vi "Finish.vi"   [LabVIEW 2015]
doc: "This VI is called just before exiting. It is expected to close I/O refnum, save collected data, etc."
uses:
  <vilib>/Rock Robotics/WPI/Utilities/WPI_GetSetVariantRefNum.vi
  navX Library v2/navX Library v2.lvlib
types:
  T1 = typedef "WPI_DigitalInputDevRef.ctl" = cluster{"DevStatus":errorcluster, "DIO Channel":T2}
  T2 = typedef "FPGA_DIOChannel.ctl" = enum8{"DIO 0", "DIO 1", "DIO 2", "DIO 3", "DIO 4", "DIO 5", "DIO 6", "DIO 7", "DIO 8", "DIO 9", "DIO MXP 0", "DIO MXP 1", "DIO MXP 2", "DIO MXP 3", "DIO MXP 4", "DIO MXP 5", "DIO MXP 6", "DIO MXP 7", "DIO MXP 8", "DIO MXP 9", "DIO MXP 10", "DIO MXP 11", "DIO MXP 12", "DIO MXP 13", "DIO MXP 14", "DIO MXP 15", "Invalid"}
  T3 = typedef "WPI_SolenoidDevRef.ctl" = cluster{"DevStatus":errorcluster, "Pneumatics Control Module":u8, "Forward Solenoid Channel":T4, "Reverse Solenoid Channel":T4}
  T4 = typedef "WPI_SolenoidChannel.ctl" = enum8{"Solenoid 0", "Solenoid 1", "Solenoid 2", "Solenoid 3", "Solenoid 4", "Solenoid 5", "Solenoid 6", "Solenoid 7", "Invalid"}
  T5 = typedef "WPI_AnalogChannelDevRef.ctl" = cluster{"DevStatus":errorcluster, "Analog Channel":T6}
  T6 = typedef "FPGA_AIChannel.ctl" = enum8{"AI 0", "AI 1", "AI 2", "AI 3", "AI MXP 0", "AI MXP 1", "AI MXP 2", "AI MXP 3", "Invalid"}
  T7 = typedef "WPI_MotorControlDeviceRef.ctl" = cluster{"DeviceStatus":errorcluster, "Type":T8, "PWM":cluster{"PWM Channel":T9, "DeadBand":T10}, "CAN":cluster{"Device Number":u8, "Control Mode":T11, "Semaphore":T12, "Max Vout":dbl, "TalonSRX Control Mode":T13}, "Invert":bool}
  T8 = typedef "WPI_MotorControlType.ctl" = enum16{"PWM", "CAN", "CANTalonSRX"}
  T9 = typedef "FPGA_DIOPWMChannel.ctl" = enum8{"PWM 0", "PWM 1", "PWM 2", "PWM 3", "PWM 4", "PWM 5", "PWM 6", "PWM 7", "PWM 8", "PWM 9", "PWM MXP 0", "PWM MXP 1", "PWM MXP 2", "PWM MXP 3", "PWM MXP 4", "PWM MXP 5", "PWM MXP 6", "PWM MXP 7", "PWM MXP 8", "PWM MXP 9", "Invalid"}
  T10 = typedef "WPI_PWMDeadband.ctl" = cluster{"Name":string, "maxPositivePwm":i32, "minPositivePwm":i32, "centerPwm":i32, "maxNegativePwm":i32, "minNegativePwm":i32, "angularRange":u16}
  T11 = typedef "WPI_CANJaguar_ControlMode.ctl" = enum8{"Percent VBus", "Current", "Speed", "Position", "Voltage"}
  T12 = typedef "Semaphore RefNum" = refnum<k1>
  T13 = typedef "WPI_CANTalonSRX_APIControlMode.ctl" = enum8{"Percent VBus", "Speed", "Position", "Slave", "Unchanged / Invalid", "Voltage Compensation", "Current", "Motion Profile"}
  T14 = typedef "WPI_JoystickDevRef.ctl" = cluster{"Device":T15}
  T15 = typedef "WPI_JoystickDeviceEnum.ctl" = enum16{"USB 0", "USB 1", "USB 2", "USB 3", "USB 4", "USB 5"}
  T16 = typedef "WPI_PotentiometerDevRef.ctl" = cluster{"DevStatus":errorcluster, "Analog Channel":T6, "Invert Output":bool}
  T17 = typedef "WPI_EncoderDevRef.ctl" = cluster{"DevStatus":errorcluster, "EncoderIndex":T18, "CounterIndex":T19, "DistancePerCount":dbl, "Decoding Type":T20}
  T18 = typedef "FPGA_EncoderIdx.ctl" = enum8{"Enc 0", "Enc 1", "Enc 2", "Enc 3", "Enc 4", "Enc 5", "Enc 6", "Enc 7", "Invalid"}
  T19 = typedef "FPGA_CounterCtrSystemIndex.ctl" = enum8{"Ctr 0", "Ctr 1", "Ctr 2", "Ctr 3", "Ctr 4", "Ctr 5", "Ctr 6", "Ctr 7", "Invalid"}
  T20 = typedef "WPI_EncoderType.ctl" = enum16{"1x", "2x", "4x"}
  T21 = typedef "WPI_CompressorDevRef.ctl" = cluster{"DevStatus":errorcluster, "Pneumatics Control Module":u8}
  T22 = typedef "navX Library v2.lvlib/Z900_navX_DeviceTypeDef.ctl" = cluster{"Interface":cluster{"Protocol":T23, "Update Rate (4Hz-60Hz)":u8, "navX Open TypeDef":variant}, "Notify Packet":refnum<notifier>, "Loop VI Refnum":refnum<vi>, "Ready to Close Occurrence Refnum":refnum<k4>}
  T23 = typedef "navX Library v2.lvlib/Z900_navX_ProtocolTypeDef.ctl" = enum16{"SERIAL", "I2C", "SPI"}
  T24 = typedef "WPI_RobotDriveDevRef.ctl" = cluster{"DevStatus":errorcluster, "Motors[]":T7[], "Square Inputs":bool, "Max Output":dbl}
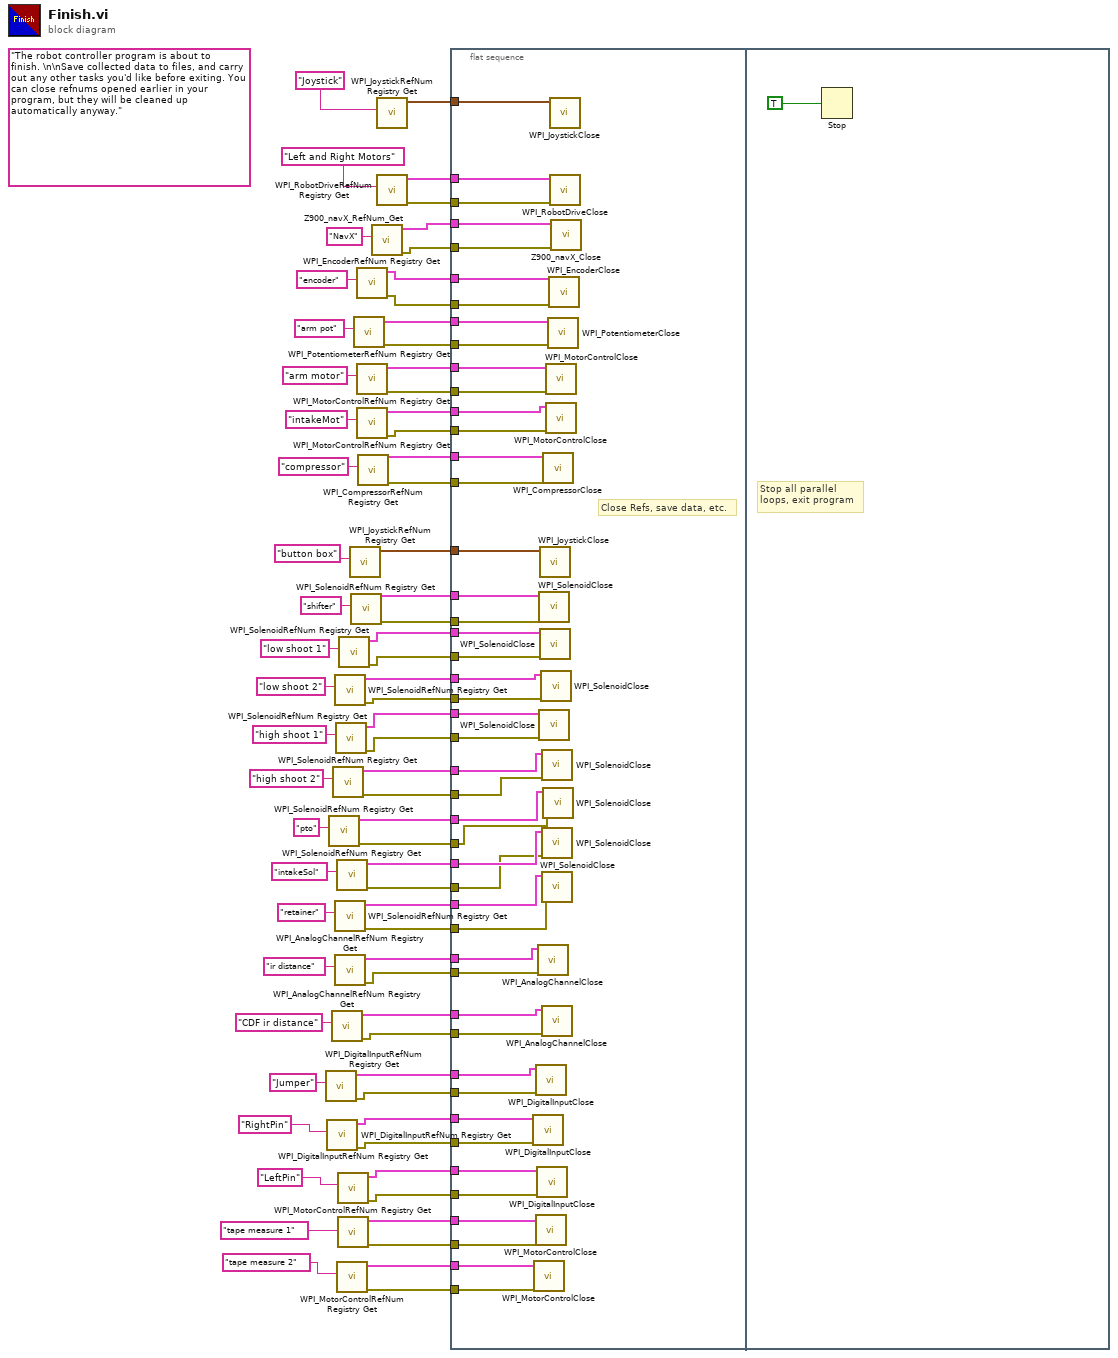
[diagram p0: block diagram]
diagram:
  (unwired) "The robot controller program is about to finish. \n\nSave collected data to files, and carry out any other tasks you'd like before exiting. You can close refnums opened earlier in your program, but they will be cleaned up automatically anyway."
  n1 = call <vilib>:"WPI_DigitalInputRefNum Registry Get.vi"("refnum name"="Jumper") -> ("error out"=w18:errorcluster, "DigitalInputDevRef"=w32:T1)  [unwired: 9 in]
  n2 = call <vilib>:"WPI_DigitalInputRefNum Registry Get.vi"("refnum name"="RightPin") -> ("error out"=w19:errorcluster, "DigitalInputDevRef"=w29:T1)  [unwired: 9 in]
  n3 = call <vilib>:"WPI_SolenoidRefNum Registry Get.vi"("refnum name"="pto") -> ("error out"=w13:errorcluster, "SolenoidDevRef"=w39:T3)  [unwired: 9 in]
  n4 = call <vilib>:"WPI_AnalogChannelRefNum Registry Get.vi"("refnum name"="CDF ir distance") -> ("error out"=w17:errorcluster, "AIDeviceRef"=w35:T5)  [unwired: 9 in]
  n5 = call <vilib>:"WPI_SolenoidRefNum Registry Get.vi"("refnum name"="high shoot 2") -> ("error out"=w12:errorcluster, "SolenoidDevRef"=w40:T3)  [unwired: 9 in]
  n6 = call <vilib>:"WPI_SolenoidRefNum Registry Get.vi"("refnum name"="low shoot 2") -> ("error out"=w10:errorcluster, "SolenoidDevRef"=w42:T3)  [unwired: 9 in]
  n7 = call <vilib>:"WPI_SolenoidRefNum Registry Get.vi"("refnum name"="retainer") -> ("error out"=w15:errorcluster, "SolenoidDevRef"=w37:T3)  [unwired: 9 in]
  n8 = call <vilib>:"WPI_AnalogChannelRefNum Registry Get.vi"("refnum name"="ir distance") -> ("error out"=w16:errorcluster, "AIDeviceRef"=w36:T5)  [unwired: 9 in]
  n9 = call <vilib>:"WPI_SolenoidRefNum Registry Get.vi"("refnum name"="high shoot 1") -> ("error out"=w11:errorcluster, "SolenoidDevRef"=w41:T3)  [unwired: 9 in]
  n10 = call <vilib>:"WPI_SolenoidRefNum Registry Get.vi"("refnum name"="intakeSol") -> ("error out"=w14:errorcluster, "SolenoidDevRef"=w38:T3)  [unwired: 9 in]
  n11 = call <vilib>:"WPI_MotorControlRefNum Registry Get.vi"("refnum name"="tape measure 2") -> ("error out"=w22:errorcluster, "MotorControlDevRef"=w23:T7)  [unwired: 9 in]
  n12 = call <vilib>:"WPI_DigitalInputRefNum Registry Get.vi"("refnum name"="LeftPin") -> ("error out"=w20:errorcluster, "DigitalInputDevRef"=w27:T1)  [unwired: 9 in]
  n13 = call <vilib>:"WPI_MotorControlRefNum Registry Get.vi"("refnum name"="tape measure 1") -> ("error out"=w21:errorcluster, "MotorControlDevRef"=w24:T7)  [unwired: 9 in]
  n14 = call <vilib>:"WPI_SolenoidRefNum Registry Get.vi"("refnum name"="low shoot 1") -> ("error out"=w9:errorcluster, "SolenoidDevRef"=w43:T3)  [unwired: 9 in]
  n15 = call <vilib>:"WPI_JoystickRefNum Registry Get.vi"("refnum name"="button box") -> ("JoystickDevRef"=w53:T14)  [unwired: 9 in, 1 out]
  n16 = call <vilib>:"WPI_SolenoidRefNum Registry Get.vi"("refnum name"="shifter") -> ("error out"=w8:errorcluster, "SolenoidDevRef"=w44:T3)  [unwired: 9 in]
  n17 = call <vilib>:"WPI_PotentiometerRefNum Registry Get.vi"("refnum name"="arm pot") -> ("error out"=w4:errorcluster, "PotDevRef"=w62:T16)  [unwired: 9 in]
  n18 = call <vilib>:"WPI_EncoderRefNum Registry Get.vi"("refnum name"="encoder") -> ("error out"=w3:errorcluster, "EncoderDevRef"=w64:T17)  [unwired: 9 in]
  n19 = call <vilib>:"WPI_MotorControlRefNum Registry Get.vi"("refnum name"="arm motor") -> ("error out"=w5:errorcluster, "MotorControlDevRef"=w60:T7)  [unwired: 9 in]
  n20 = call <vilib>:"WPI_MotorControlRefNum Registry Get.vi"("refnum name"="intakeMot") -> ("error out"=w6:errorcluster, "MotorControlDevRef"=w57:T7)  [unwired: 9 in]
  n21 = call <vilib>:"WPI_CompressorRefNum Registry Get.vi"("refnum name"="compressor") -> ("error out"=w7:errorcluster, "CompressorDevRef"=w55:T21)  [unwired: 9 in]
  n22 = call "Z900_navX_RefNum_Get.vi"("refnum name"="NavX") -> ("error out"=w2:errorcluster, "navX Device"=w66:T22)  [unwired: 9 in]
  n23 = call <vilib>:"WPI_JoystickRefNum Registry Get.vi"("refnum name"="Joystick") -> ("JoystickDevRef"=w67:T14)  [unwired: 1 in, 9 out]
  n24 = call <vilib>:"WPI_RobotDriveRefNum Registry Get.vi"("refnum name"="Left and Right Motors") -> ("error out"=w1:errorcluster, "RobotDriveDevRef"=w68:T24)  [unwired: 1 in, 8 out]
  n25 = flat-sequence {
    tunnel: w68 -> [w116]
    tunnel: w67 -> [w115]
    tunnel: w66 -> [w114]
    tunnel: w64 -> [w113]
    tunnel: w62 -> [w112]
    tunnel: w60 -> [w111]
    tunnel: w57 -> [w110]
    tunnel: w55 -> [w109]
    tunnel: w53 -> [w108]
    tunnel: w44 -> [w107]
    tunnel: w43 -> [w106]
    tunnel: w42 -> [w105]
    tunnel: w41 -> [w104]
    tunnel: w40 -> [w103]
    tunnel: w39 -> [w102]
    tunnel: w38 -> [w101]
    tunnel: w37 -> [w100]
    tunnel: w36 -> [w99]
    tunnel: w35 -> [w98]
    tunnel: w32 -> [w97]
    tunnel: w29 -> [w96]
    tunnel: w27 -> [w95]
    tunnel: w24 -> [w94]
    tunnel: w23 -> [w93]
    tunnel: w22 -> [w92]
    tunnel: w21 -> [w91]
    tunnel: w20 -> [w90]
    tunnel: w19 -> [w89]
    tunnel: w18 -> [w88]
    tunnel: w17 -> [w87]
    tunnel: w16 -> [w86]
    tunnel: w15 -> [w85]
    tunnel: w14 -> [w84]
    tunnel: w13 -> [w83]
    tunnel: w12 -> [w82]
    tunnel: w11 -> [w81]
    tunnel: w10 -> [w80]
    tunnel: w9 -> [w79]
    tunnel: w8 -> [w78]
    tunnel: w7 -> [w77]
    tunnel: w6 -> [w76]
    tunnel: w5 -> [w75]
    tunnel: w4 -> [w74]
    tunnel: w3 -> [w73]
    tunnel: w2 -> [w72]
    tunnel: w1 -> [w71]
    frame #0 {
      # "Close Refs, save data, etc."
      n26 = call <vilib>:"WPI_DigitalInputClose.vi"("error in (no error)"=w89, "DigitalInputDevRef"=w96) -> ()  [unwired: 9 in, 1 out]
      n27 = call <vilib>:"WPI_MotorControlClose.vi"("error in (no error)"=w92, "MotorControlDevRef"=w93) -> ()  [unwired: 9 in, 1 out]
      n28 = call <vilib>:"WPI_DigitalInputClose.vi"("error in (no error)"=w88, "DigitalInputDevRef"=w97) -> ()  [unwired: 9 in, 1 out]
      n29 = call <vilib>:"WPI_MotorControlClose.vi"("error in (no error)"=w91, "MotorControlDevRef"=w94) -> ()  [unwired: 9 in, 1 out]
      n30 = call <vilib>:"WPI_DigitalInputClose.vi"("error in (no error)"=w90, "DigitalInputDevRef"=w95) -> ()  [unwired: 9 in, 1 out]
      n31 = call <vilib>:"WPI_AnalogChannelClose.vi"("error in (no error)"=w86, "AIDeviceRef"=w99) -> ()  [unwired: 9 in, 1 out]
      n32 = call <vilib>:"WPI_SolenoidClose.vi"("error in (no error)"=w78, "SolenoidDevRef"=w107) -> ()  [unwired: 9 in, 1 out]
      n33 = call <vilib>:"WPI_SolenoidClose.vi"("error in (no error)"=w81, "SolenoidDevRef"=w104) -> ()  [unwired: 9 in, 1 out]
      n34 = call <vilib>:"WPI_JoystickClose.vi"("JoystickDevRef"=w108) -> ()  [unwired: 11 in]
      n35 = call <vilib>:"WPI_SolenoidClose.vi"("error in (no error)"=w79, "SolenoidDevRef"=w106) -> ()  [unwired: 9 in, 1 out]
      n36 = call <vilib>:"WPI_SolenoidClose.vi"("error in (no error)"=w80, "SolenoidDevRef"=w105) -> ()  [unwired: 9 in, 1 out]
      n37 = call <vilib>:"WPI_SolenoidClose.vi"("error in (no error)"=w82, "SolenoidDevRef"=w103) -> ()  [unwired: 9 in, 1 out]
      n38 = call <vilib>:"WPI_SolenoidClose.vi"("error in (no error)"=w84, "SolenoidDevRef"=w101) -> ()  [unwired: 9 in, 1 out]
      n39 = call <vilib>:"WPI_SolenoidClose.vi"("error in (no error)"=w85, "SolenoidDevRef"=w100) -> ()  [unwired: 9 in, 1 out]
      n40 = call <vilib>:"WPI_AnalogChannelClose.vi"("error in (no error)"=w87, "AIDeviceRef"=w98) -> ()  [unwired: 9 in, 1 out]
      n41 = call <vilib>:"WPI_CompressorClose.vi"("error in (no error)"=w77, "CompressorDevRef"=w109) -> ()  [unwired: 9 in, 1 out]
      n42 = call <vilib>:"WPI_SolenoidClose.vi"("error in (no error)"=w83, "SolenoidDevRef"=w102) -> ()  [unwired: 9 in, 1 out]
      n43 = call <vilib>:"WPI_MotorControlClose.vi"("error in (no error)"=w75, "MotorControlDevRef"=w111) -> ()  [unwired: 9 in, 1 out]
      n44 = call <vilib>:"WPI_MotorControlClose.vi"("error in (no error)"=w76, "MotorControlDevRef"=w110) -> ()  [unwired: 9 in, 1 out]
      n45 = call <vilib>:"WPI_PotentiometerClose.vi"("error in"=w74, "PotDevRef"=w112) -> ()  [unwired: 9 in, 1 out]
      n46 = call <vilib>:"WPI_EncoderClose.vi"("error in (no error)"=w73, "EncoderDevRef"=w113) -> ()  [unwired: 9 in, 1 out]
      n47 = call <vilib>:"WPI_JoystickClose.vi"("JoystickDevRef"=w115) -> ()  [unwired: 11 out]
      n48 = call <vilib>:"WPI_RobotDriveClose.vi"("error in (no error)"=w71, "RobotDriveDevRef"=w116) -> ()  [unwired: 10 out]
      n49 = call "Z900_navX_Close.vi"("error in (no error)"=w72, "navX Device"=w114) -> ()  [unwired: 9 in, 1 out]
    }
    frame #1 {
      # "Stop all parallel\nloops, exit program"
      n50 = Stop(stop? (T)=TRUE ("Quit")) -> ()
    }
  }
